vi "View整体图.vi"() -> ()   [LabVIEW 2014]
panel:
  in  "Background":bool
  in  "Arm":bool
  in  "Apps":bool
  in  "World clock":bool
  in  "Windows":bool
  in  "Viewer":bool
  in  "View all":bool
  in  "Tree":bool
  in  "Thumbnail":bool
  in  "Text":bool
  in  "Terminal":bool
  in  "Stylesheet":bool
  in  "Style":bool
  in  "Splash":bool
  in  "Snap shot":bool
  in  "Signature":bool
  in  "Sidetree":bool
  in  "Side":bool
  in  "Screensaver":bool
  in  "Remove":bool
  in  "Remove tab":bool
  in  "Reduce":bool
  in  "Rebuild":bool
  in  "Properties":bool
  in  "Presenter":bool
  in  "Photo":bool
  in  "Pdf viewer":bool
  in  "Pager":bool
  in  "Open":bool
  in  "New":bool
  in  "New tab":bool
  in  "New raised tab":bool
  in  "Multicolumn":bool
  in  "Magnify":bool
  in  "Mag+":bool
  in  "Mag-":bool
  in  "Mag":bool
  in  "Mag fit":bool
  in  "List":bool
  in  "Index imager":bool
  in  "Icons":bool
  in  "Icon":bool
  in  "Icon themes":bool
  in  "Horizontal":bool
  in  "Fullscreen":bool
  in  "Fit screen":bool
  in  "Finder":bool
  in  "Edit menu":bool
  in  "Duplicate tab":bool
  in  "Dos":bool
  in  "Display":bool
  in  "Develop":bool
  in  "Detailed":bool
  in  "Desktop":bool
  in  "Create":bool
  in  "Console":bool
  in  "Colors":bool
  in  "Choose":bool
  in  "Bottom":bool
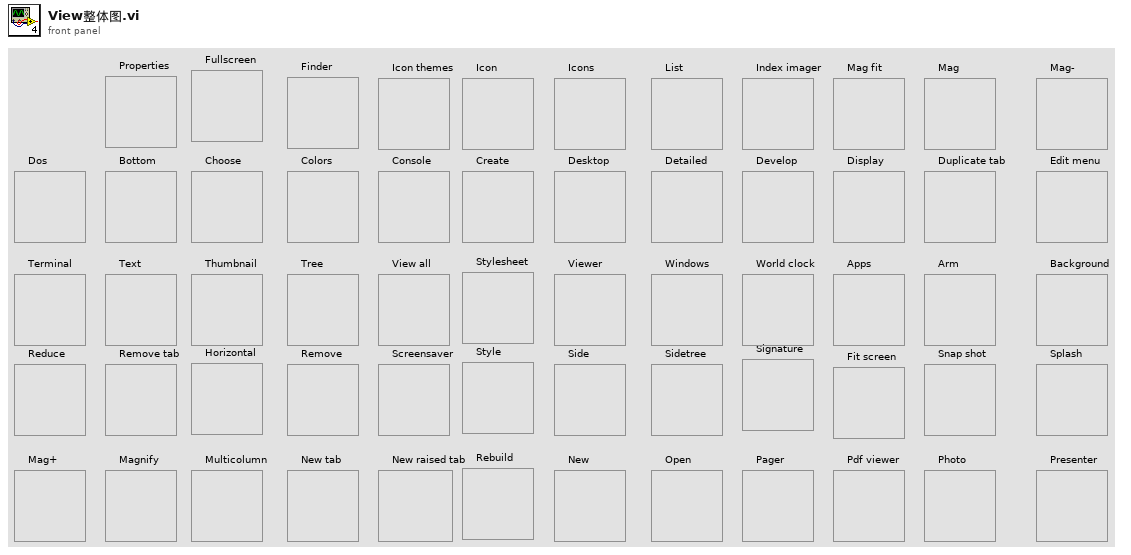
[diagram p1: front panel]
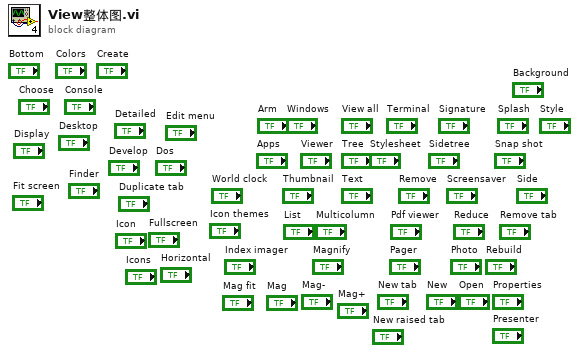
[diagram p0: block diagram]
diagram:
